vi "Update Measurements.vi"(7 "Update OUR":bool, 8 "error in (no error)":errorcluster, 9 "Control (aeration)":bool, 10 "So_measured":dbl, 11 "Model_Predictor in":refnum<class "Model_Predictor.lvclass">) -> (0 "error out":errorcluster, 3 "Model_Predictor out":refnum<class "Model_Predictor.lvclass">)   [LabVIEW 2021, in "MBPOnOff_Controller.lvlib" / "Model_Predictor.lvclass"]
uses:
  Model_Predictor.lvclass
  Model_Predictor.lvclass/Model_Predictor.ctl
  OUR_Monitor/OUR_Monitor.lvclass/OUR_Monitor.ctl
  OUR_Monitor/Read OUR.vi
  OUR_Monitor/OUR_Monitor.lvclass
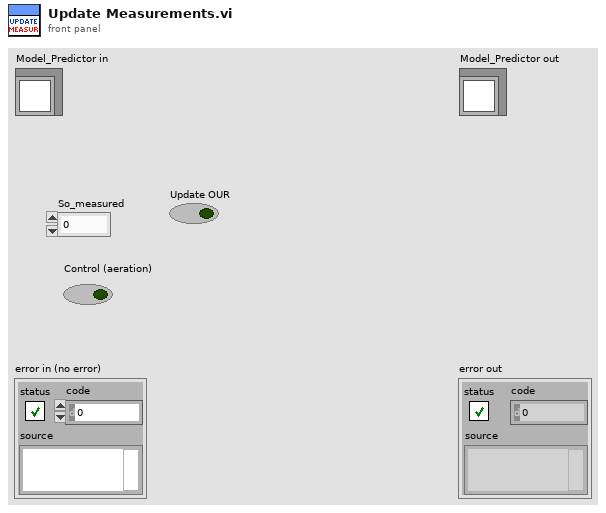
[diagram p1: front panel]
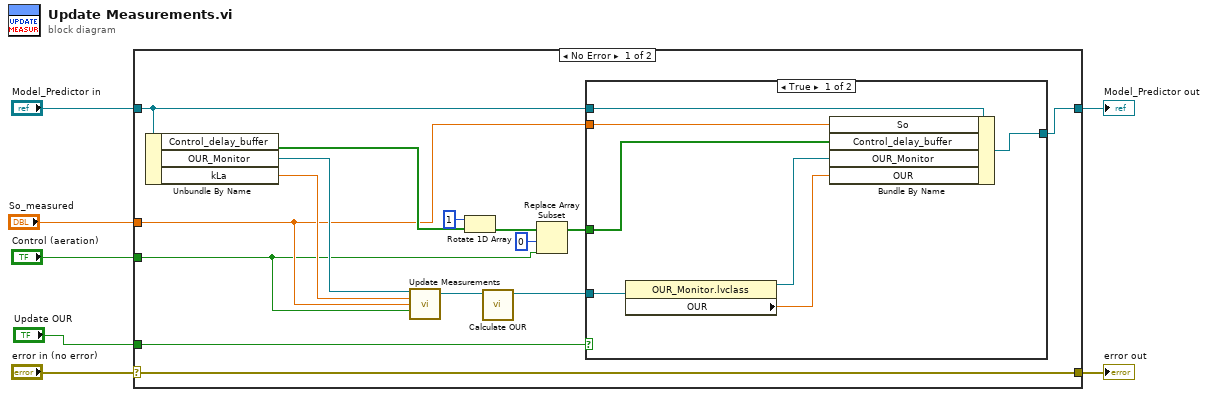
[diagram p0: block diagram]
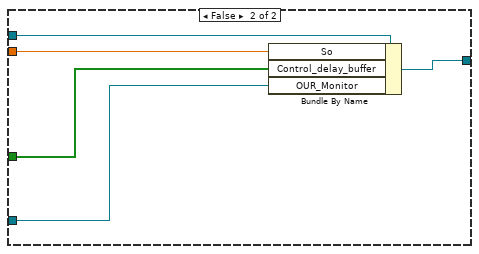
[diagram p2: hidden frame]
diagram:
  n1 = case shown="No Error" "error in (no error)" {
    selector: "error in (no error)" -> [w22 w36]
    tunnel: [w22 w36] -> w6
    tunnel: [w21 w35] -> w4
    tunnel: "Model_Predictor in" -> [w20 w35]
    tunnel: "So_measured" -> [w12 _]
    tunnel: "Control (aeration)" -> [w11 _]
    tunnel: "Update OUR" -> [w9 _]
    frame No Error {
      n2 = Unbundle By Name(w20) -> ("Control_delay_buffer"=w19:bool[], "OUR_Monitor"=w14:refnum<class "OUR_Monitor.lvclass">, "kLa"=w13:dbl)
      n3 = call "Update Measurements.vi"("OUR Monitor in"=w14, "kla"=w13, "So"=w12, "CV"=w11) -> ("OUR Monitor out"=w10:refnum<class "OUR_Monitor.lvclass">)  [unwired: 10 in, 1 out]
      n4 = Rotate 1D Array(1:w19, 2:1 ("n")) -> (0:w17:bool[])
      n5 = call "Calculate OUR.vi"("OUR_Monitor in"=w10) -> ("OUR_Monitor out"=w8:refnum<class "OUR_Monitor.lvclass">)  [unwired: 9 in, 1 out]
      n6 = Replace Array Subset(array=w17, new element=w11, index=0) -> (w15:bool[])
      n7 = case shown="True" w9 {
        tunnel: [w29 w34] -> w21
        tunnel: w20 -> [w28 w33]
        tunnel: w15 -> [w27 w32]
        tunnel: w12 -> [w26 w31]
        tunnel: w8 -> [w25 w30]
        frame True {
          n8 = property class="OUR_Monitor.lvclass"(reference=w25) -> (reference out=w23:refnum<class "OUR_Monitor.lvclass">, "OUR"=w24:dbl)  [unwired: 1 in, 1 out]
          n9 = Bundle By Name(cluster=w28, "So"=w26, "Control_delay_buffer"=w27, "OUR_Monitor"=w23, "OUR"=w24) -> (w29:refnum<class "Model_Predictor.lvclass">)
        }
        frame False {
          n10 = Bundle By Name(cluster=w33, "So"=w31, "Control_delay_buffer"=w32, "OUR_Monitor"=w30) -> (w34:refnum<class "Model_Predictor.lvclass">)
        }
      }
    }
    frame Error {
    }
  }
  "error out" <- w6
  "Model_Predictor out" <- w4
